vi "pb_inst_pbonly.vi"(8 "error in (no error)":errorcluster, 10 "PB Instruction":T1={"Instruct Data"=0, "Op Code"=0, "Flags"=[FALSE, FALSE, FALSE, FALSE, FALSE, FALSE, FALSE, FALSE, FALSE, FALSE, FALSE, FALSE, FALSE, FALSE, FALSE, FALSE, FALSE, FALSE, FALSE, FALSE, FALSE, FALSE, FALSE, FALSE], "Comments"="", "Time"=0.016675} {"Time" format="%.3p"; "Op Code" items=["Continue", "Stop", "Loop", "End Loop", "JSR", "RTS", "Branch", "Long Delay", "Wait"]}, 11 "path in":path=path "C:/Program Files/SpinCore/SpinAPI/dll/spinapi.dll") -> (0 "error out":errorcluster, 3 "path out":path)   [LabVIEW 2016]
panel:
  out "inst":i32
  # "1"
  # "2"
  # "3"
  # "4"
  # "5"
  # "6"
  # "7"
  # "8"
  # "9"
  # "10"
  # "11"
  # "12"
  # "13"
  # "14"
  # "15"
  # "16"
  # "17"
  # "18"
  # "19"
  # "20"
  # "21"
  # "22"
  # "23"
  # "24"
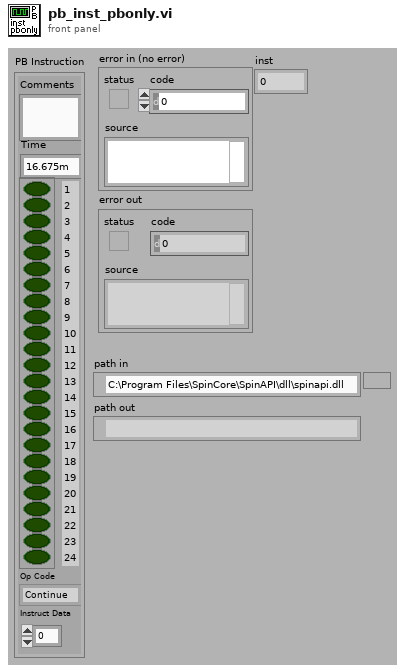
[diagram p1: front panel]
types:
  T1 = cluster{"Instruct Data":i32, "Op Code":i32, "Flags":bool[], "Comments":string, "Time":dbl}
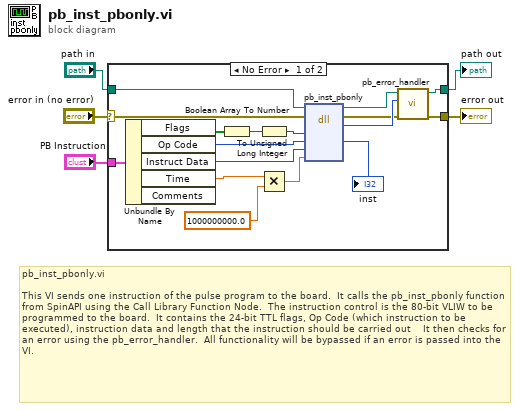
[diagram p0: block diagram]
diagram:
  # "pb_inst_pbonly.vi\n\nThis VI sends one instruction of the pulse program to the board.  It calls the pb_inst_pbonly function from SpinAPI using the Call Library Function Node.  The instruction control is the 80-bit VLIW to be programmed to the board.  It contains the 24-bit TTL flags, Op Code (which instruction to be executed), instruction data and length that the instruction should be carried out    It then checks for an error using the pb_error_handler.  All functionality will be bypassed if an error is passed into the VI."
  n1 = case shown="No Error" "error in (no error)" {
    selector: "error in (no error)" -> [w12 w24]
    tunnel: "PB Instruction" -> [w22 _]
    tunnel: [w7 w24] -> w4
    tunnel: "path in" -> [w11 w23]
    tunnel: [w8 w23] -> w1
    frame No Error {
      n2 = Unbundle By Name(w22) -> ("Flags"=w21:bool[], "Op Code"=w18:i32, "Instruct Data"=w17:i32, "Time"=w15:dbl)  [unwired: 1 out]
      n3 = Boolean Array To Number(Boolean array=w21) -> (number=w20:u32)
      n4 = To Unsigned Long Integer(number=w20) -> (unsigned 32bit integer=w19:u32)
      n5 = Multiply(x=w15, y=1000000000.0) -> (x*y=w13:dbl)
      n6 = dll-call lib="C:/Program Files/SpinCore/SpinAPI/dll/spinapi.dll" fn="pb_inst_pbonly"(path in=w11, error in=w12, "flags"=w19, "inst"=w18, "inst_data"=w17, "length"=w13) -> (path out=w10:path, error out=w9:errorcluster, "return type"=w16:i32, "inst"=→"inst":i32)  [unwired: 4 in]
      n7 = call "pb_error_handler.vi"("error in (no error)"=w9, "return code"=w16, "path in"=w10) -> ("error out"=w7:errorcluster, "path out"=w8:path)  [unwired: 7 out]
    }
    frame Error {
    }
  }
  "error out" <- w4
  "path out" <- w1
